vi "AFG Config DC Voltage.vi"(8 "error in (no error)":errorcluster, 10 "DC Amplitude":dbl, 11 "Actor_AFG in":refnum<class "Actor_AFG.lvclass">) -> (0 "error out":errorcluster, 3 "Actor_AFG out":refnum<class "Actor_AFG.lvclass">)   [LabVIEW 2020, in "Actor_AFG.lvlib" / "Actor_AFG.lvclass"]
uses:
  Actor_AFG.lvclass
  C:/Program Files/National Instruments/LabVIEW 2020/vi.lib/ActorFramework/Actor/Actor.lvclass
  AFG_Event.ctl
  Actor_AFG.lvclass/Actor_AFG.ctl
  <vilib>/ActorFramework/Actor/Actor.lvclass/Actor.ctl
  <vilib>/ActorFramework/Actor/Actor.lvclass
  <instrlib>/Tektronix AFG 3000 Series/Tektronix AFG 3000 Series.lvlib
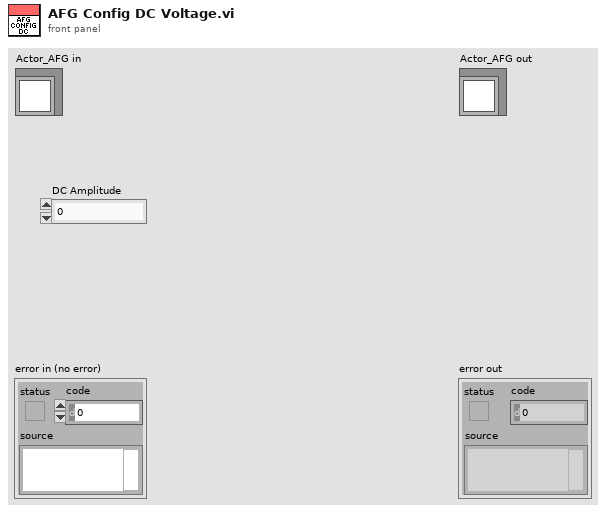
[diagram p1: front panel]
types:
  T1 = typedef "Actor_AFG.lvlib/Actor_AFG.lvclass/AFG_Event.ctl" = enum16{"General Event", "Inited", "Output", "Waveform Set", "DC Configured", "Cycle End", "Error"}
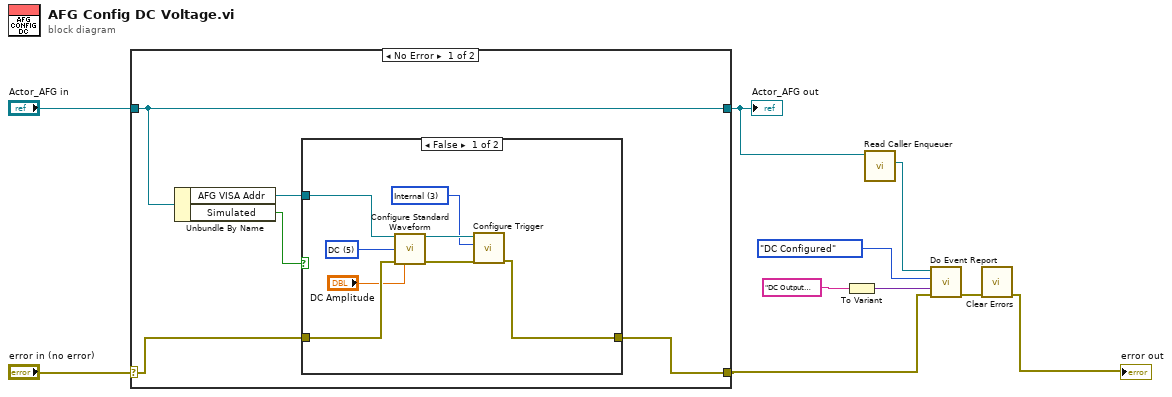
[diagram p0: block diagram]
diagram:
  n1 = case shown="No Error" "error in (no error)" {
    selector: "error in (no error)" -> [w15 w26]
    tunnel: [w11 w26] -> w3
    tunnel: [w14 w25] -> w2
    tunnel: "Actor_AFG in" -> [w14 w25]
    frame No Error {
      n2 = Unbundle By Name(w14) -> ("AFG VISA Addr"=w13:refnum<visa-resource-name>, "Simulated"=w12:bool)
      n3 = case shown="False" w12 {
        tunnel: w15 -> [w22 w24]
        tunnel: w13 -> [w21 _]
        tunnel: [w17 w24] -> w11
        frame False {
          w18 = u16 3 items=["Internal"=3, "External"=1] ("Trigger Source (3:Internal)")
          w23 = u16 5 items=["Sine", "Square", "Pulse", "Ramp", "Noise", "DC", "Sin(x)/x", "Gaussian", "Lorentz", "Exponential Rise", "Exponential Decay", "Haversine"] ("Waveform Function (0: Sine)")
          n4 = call <instrlib>:"Configure Standard Waveform.vi"("VISA resource name"=w21, "Waveform Function (0: Sine)"=w23, "error in (no error)"=w22, "DC Offset (0.00 V)"="DC Amplitude") -> ("VISA resource name out"=w20:refnum<visa-resource-name>, "error out"=w19:errorcluster)  [unwired: 10 in]
          n5 = call <instrlib>:"Configure Trigger.vi"("error in (no error)"=w19, "Trigger Source (3:Internal)"=w18, "VISA resource name"=w20) -> ("error out"=w17:errorcluster)  [unwired: 7 in, 1 out]
        }
        frame True {
        }
      }
    }
    frame Error {
    }
  }
  "Actor_AFG out" <- w2
  n6 = To Variant(anything="DC Output configured successful") -> (Variant=w6:variant)
  n7 = call <vilib>:"Read Caller Enqueuer.vi"("Actor"=w2) -> ("Caller Enqueuer"=w8:refnum<class "Message Enqueuer.lvclass">)  [unwired: 10 in]
  n8 = call "Do Event Report.vi"("error in (no error)"=w3, "Event Data"=w6, "Report Events"=AFG_Event."DC Configured", "Caller Enqueuer"=w8) -> ("error out"=w7:errorcluster)  [unwired: 6 in, 1 out]
  n9 = call <vilib>:"Clear Errors.vi"("error in (no error)"=w7) -> ("error out"=→"error out":errorcluster)  [unwired: 5 in, 1 out]
